vi "FP add waypoints.vi"(2 "error in":errorcluster, 3 "MDF Control":T1(array[cluster]), 4 "Image In":T2) -> (0 "error out":errorcluster, 1 "Image Out":T2)   [LabVIEW 2014]
doc: "This vi will overlay the waypoints created in the Mission Definition File onto the pool image."
uses:
  <vilib>/vision/Image Controls.llb/IMAQ Image.ctl
panel:
  out "size(s)":i32
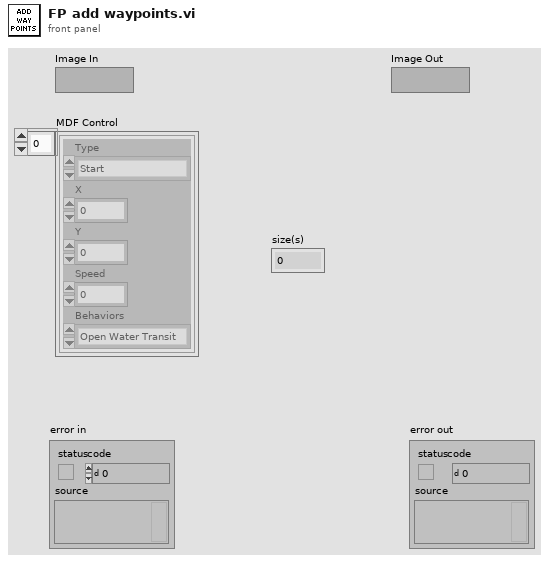
[diagram p1: front panel]
types:
  T1 = cluster{"Type":enum16{"Start", "Waypoint", "End"}, "X":i32, "Y":i32, "Speed":i32, "Behaviors":enum16{"Open Water Transit", "P-Wall Follow", "S-Wall Follow", "Dock"}}[]
  T2 = typedef "IMAQ Image.ctl" = refnum<image>
  T3 = cluster{"Desired Font (Application)":enum16{"User-specified Font", "Application Font", "System Font", "Dialog Font"}, "[User-specified Font]":cluster{"Font Name":string, "Size":i16, "Strikeout?":bool, "Italic?":bool, "Underline?":bool, "Outline?":bool, "Shadow?":bool, "Bold?":bool, "Rotation Angle":dbl}, "Horizontal Alignment":i16, "Vertical Alignment":i16}
  T4 = cluster{"Type":enum16{"Start", "Waypoint", "End"}, "X":i32, "Y":i32, "Speed":i32, "Behaviors":enum16{"Open Water Transit", "P-Wall Follow", "S-Wall Follow", "Dock"}}
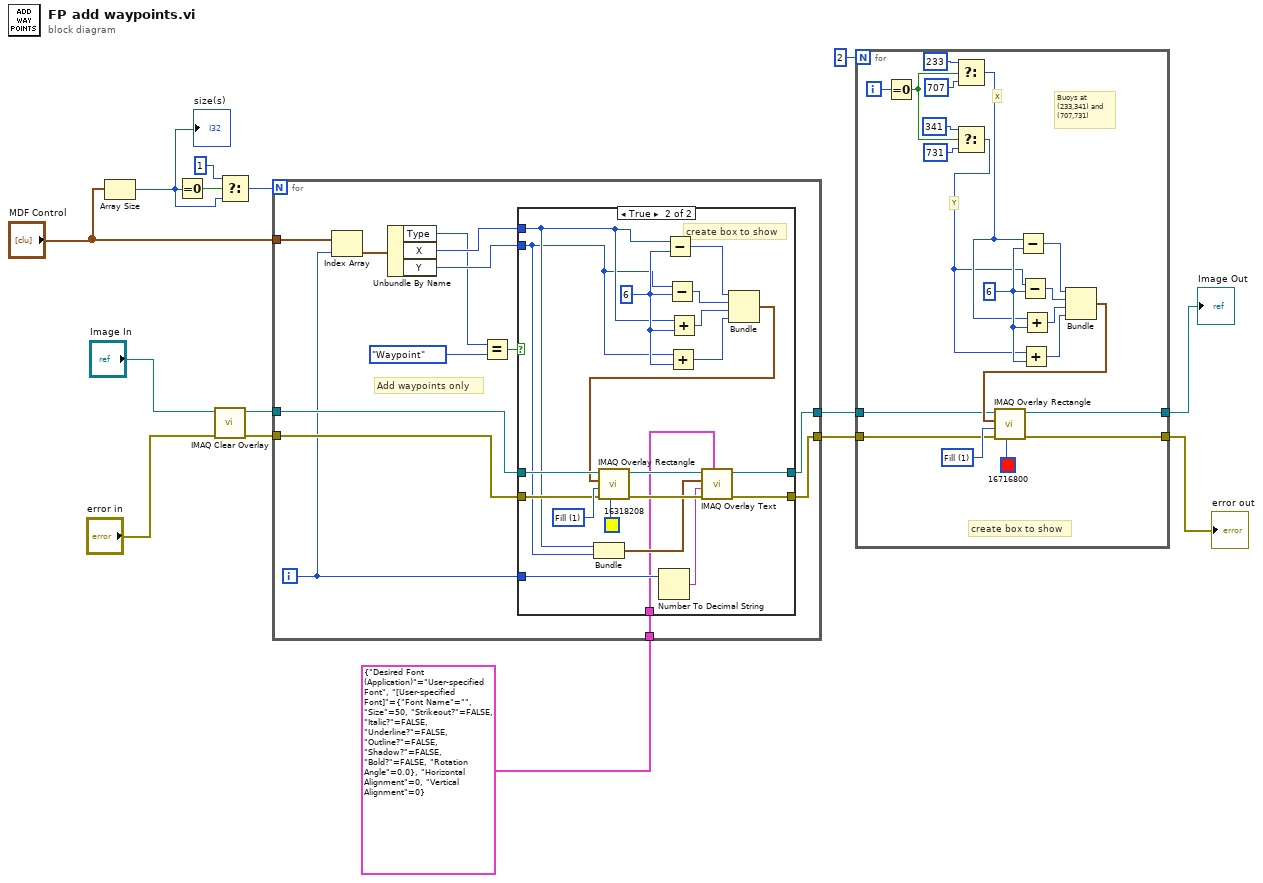
[diagram p0: block diagram]
diagram:
  n1 = Array Size(array="MDF Control") -> (size(s)=w8:i32)
  "size(s)" <- w8
  n2 = Equal To 0?(x=w8) -> (x = 0?=w11:bool)
  n3 = call "IMAQ Clear Overlay"("error in (no error)"="error in", "Image"="Image In") -> ("error out"=w14:errorcluster, "Image Out"=w12:T2)  [unwired: 8 in]
  n4 = Select(t=1, s=w11, f=w8) -> (s? t:f=w9:i32)
  n5 = for {
    N: w9 -> [_]
    tunnel: [w28] -> w6
    tunnel: [w27] -> w4
    tunnel: w14 -> [w26]
    tunnel: w12 -> [w25]
    tunnel: "MDF Control" -> [w24]
    tunnel: T3 {"Desired Font (Application)"=enum."User-specified Font", "[User-specified Font]"={"Font Name"="", "Size"=50, "Strikeout?"=FALSE, "Italic?"=FALSE, "Underline?"=FALSE, "Outline?"=FALSE, "Shadow?"=FALSE, "Bold?"=FALSE, "Rotation Angle"=0.0}, "Horizontal Alignment"=0, "Vertical Alignment"=0} ("Font, Size & Style") -> [w16]
    i -> [w17]
    # "Add waypoints only"
    n6 = Index Array(array=w24, index=w17) -> (element=w23:T4)
    n7 = Unbundle By Name(w23) -> ("Type"=w19:enum16{"Start", "Waypoint", "End"}, "X"=w22:i32, "Y"=w21:i32)
    n8 = Equal?(x=w19, y=enum16{"Start", "Waypoint", "End"}."Waypoint" ("Type")) -> (x = y?=w20:bool)
    n9 = case shown="True" w20 {
      tunnel: [w30 w39] -> w28
      tunnel: [w29 w37] -> w27
      tunnel: w26 -> [w29 w48]
      tunnel: w25 -> [w30 w47]
      tunnel: w22 -> [_ w34]
      tunnel: w21 -> [_ w33]
      tunnel: w17 -> [_ w36]
      tunnel: w16 -> [_ w31]
      frame False {
      }
      frame True {
        w46 = 6
        w49 = u32 1 items=["Frame", "Fill", "Highlight"] ("Drawing Mode (Frame)")
        # "create box to show"
        n10 = Bundle("X"=w34, "Y"=w33) -> (w32:cluster{"X":i32, "Y":i32})  [unwired: 1 in]
        n11 = Number To Decimal String(number=w36) -> (decimal integer string=w35:string)  [unwired: 1 in]
        n12 = Subtract(x=w34, y=w46) -> (x-y=w45:i32)
        n13 = Subtract(x=w33, y=w46) -> (x-y=w44:i32)
        n14 = Add(x=w33, y=w46) -> (x+y=w42:i32)
        n15 = Add(x=w34, y=w46) -> (x+y=w43:i32)
        n16 = Bundle(w45, w44, w43, w42) -> (w41:cluster{i32, i32, i32, i32})  [unwired: 1 in]
        n17 = call "IMAQ Overlay Rectangle"("Color"=u32 16318208, "error in (no error)"=w48, "Drawing Mode (Frame)"=w49, "Rectangle"=w41, "Image"=w47) -> ("error out"=w38:errorcluster, "Image Out"=w40:T2)  [unwired: 5 in]
        n18 = call "IMAQ Overlay Text"("Font, Size & Style"=w31, "error in (no error)"=w38, "String"=w35, "Origin"=w32, "Image"=w40) -> ("error out"=w37:errorcluster, "Image Out"=w39:T2)  [unwired: 5 in]
      }
    }
  }
  n19 = for {
    N: 2 -> [_]
    tunnel: w6 -> [w62]
    tunnel: [w51] -> w5
    tunnel: w4 -> [w61]
    tunnel: [w52] -> w3
    i -> [w53]
    w68 = 6
    w69 = u32 1 items=["Frame", "Fill", "Highlight"] ("Drawing Mode (Frame)")
    # "Buoys at \n(233,341) and \n(707,731)"
    # "Y"
    # "X"
    # "create box to show"
    n20 = Equal To 0?(x=w53) -> (x = 0?=w60:bool)
    n21 = Select(t=233, s=w60, f=707 ("t")) -> (s? t:f=w55:i32)
    n22 = Select(t=341, s=w60, f=731 ("t")) -> (s? t:f=w54:i32)
    n23 = Subtract(x=w55, y=w68) -> (x-y=w67:i32)
    n24 = Subtract(x=w54, y=w68) -> (x-y=w66:i32)
    n25 = Add(x=w54, y=w68) -> (x+y=w64:i32)
    n26 = Add(x=w55, y=w68) -> (x+y=w65:i32)
    n27 = Bundle(w67, w66, w65, w64) -> (w63:cluster{i32, i32, i32, i32})  [unwired: 1 in]
    n28 = call "IMAQ Overlay Rectangle"("Color"=u32 16716800, "error in (no error)"=w61, "Drawing Mode (Frame)"=w69, "Rectangle"=w63, "Image"=w62) -> ("error out"=w52:errorcluster, "Image Out"=w51:T2)  [unwired: 5 in]
  }
  "Image Out" <- w5
  "error out" <- w3
